vi "Temp ctrl - Read temp and stp.vi"(5 "Error In":errorcluster, 8 "Temp handle":T1={"Connected"=FALSE, "Temp ctrl"={"Gain (P)"=0.0, "Reset (I)"=0.0, "Rate (D)"=0.0, "Stabilization rate"=0.0, "Stabilization delta"=0.0, "Type"=enum."Lake Shore 325", "Custom temp ctrl"={"VISA resource name"=""}, "Lakeshore 325"={"VISA name"="", "Loop"=0, "Heater Range"=1, "Heater Resistance"=0, "Sample sensor"=0, "Fast sensor"=0, "Slow sensor"=0}, "Lakeshore 331"={"VISA name"="", "Loop"=1, "Heater Range"=0, "Sample sensor"=0, "Fast sensor"=0, "Slow sensor"=0}, "Lakeshore 332"={"VISA name"="", "Loop"=1, "Heater Range"=0, "Sample sensor"=0, "Fast sensor"=0, "Slow sensor"=0}, "Lakeshore 335"={"VISA name"="", "Loop"=1, "Sample sensor"=0, "Fast sensor"=0, "Slow sensor"=0}}} {"Temp ctrl"."Lakeshore 335"."Slow sensor" items=["A", "B"]; "Temp ctrl"."Lakeshore 335"."Fast sensor" items=["A", "B"]; "Temp ctrl"."Lakeshore 335"."Sample sensor" items=["A", "B"]; "Temp ctrl"."Lakeshore 335"."Loop" items=["Loop 1"=1, "Loop 2"=2]; "Temp ctrl"."Lakeshore 332"."Slow sensor" items=["A", "B"]; "Temp ctrl"."Lakeshore 332"."Fast sensor" items=["A", "B"]; "Temp ctrl"."Lakeshore 332"."Sample sensor" items=["A", "B"]; "Temp ctrl"."Lakeshore 332"."Heater Range" items=["Off", "Low (0.5W)", "Med (5W)", "High (50W)"]; "Temp ctrl"."Lakeshore 332"."Loop" items=["Loop 1", "Loop 2"]; "Temp ctrl"."Lakeshore 331"."Slow sensor" items=["A", "B"]; "Temp ctrl"."Lakeshore 331"."Fast sensor" items=["A", "B"]; "Temp ctrl"."Lakeshore 331"."Sample sensor" items=["A", "B"]; "Temp ctrl"."Lakeshore 331"."Heater Range" items=["Off", "Low (0.5W)", "Med (5W)", "High (50W)"]; "Temp ctrl"."Lakeshore 331"."Loop" items=["Loop 1", "Loop 2"]; "Temp ctrl"."Lakeshore 325"."Slow sensor" items=["A", "B"]; "Temp ctrl"."Lakeshore 325"."Fast sensor" items=["A", "B"]; "Temp ctrl"."Lakeshore 325"."Sample sensor" items=["A", "B"]; "Temp ctrl"."Lakeshore 325"."Heater Resistance" items=["25 Ohm"=1, "50 Ohm"=2]; "Temp ctrl"."Lakeshore 325"."Heater Range" items=["Off", "Low (loop 1) or On (loop 2)", "High (loop 1)"]; "Temp ctrl"."Lakeshore 325"."Loop" items=["Loop 1"=1, "Loop 2"=2]}) -> (0 "Error Out":errorcluster, 1 "Slow changing temp":dbl[unit], 2 "Fast changing temp":dbl[unit], 3 "Sample temperature":dbl[unit], 4 "Setpoint":dbl[unit])   [LabVIEW 2019]
doc: "Reads current temperatures and temperature setpoint from the temperature controller"
uses:
  Type defs/Temp handle Type Def.ctl
  Type defs/Temp ctrl Type Def.ctl
  Custom devices/Custom temp ctrl settings.ctl
  <instrlib>/Lake Shore 325/Public/Data/Sensor Data (Single Reading).vi
  <instrlib>/Lake Shore 335/Public/Data/Sensor Data (Single Reading).vi
  <instrlib>/Lake Shore 325/Lake Shore 325.lvlib
  <instrlib>/Lake Shore Cryotronics 331/Lake Shore Cryotronics 331.lvlib
  <instrlib>/Lake Shore Cryotronics 332/Lake Shore Cryotronics 332.lvlib
  <instrlib>/Lake Shore 335/Lake Shore 335.lvlib
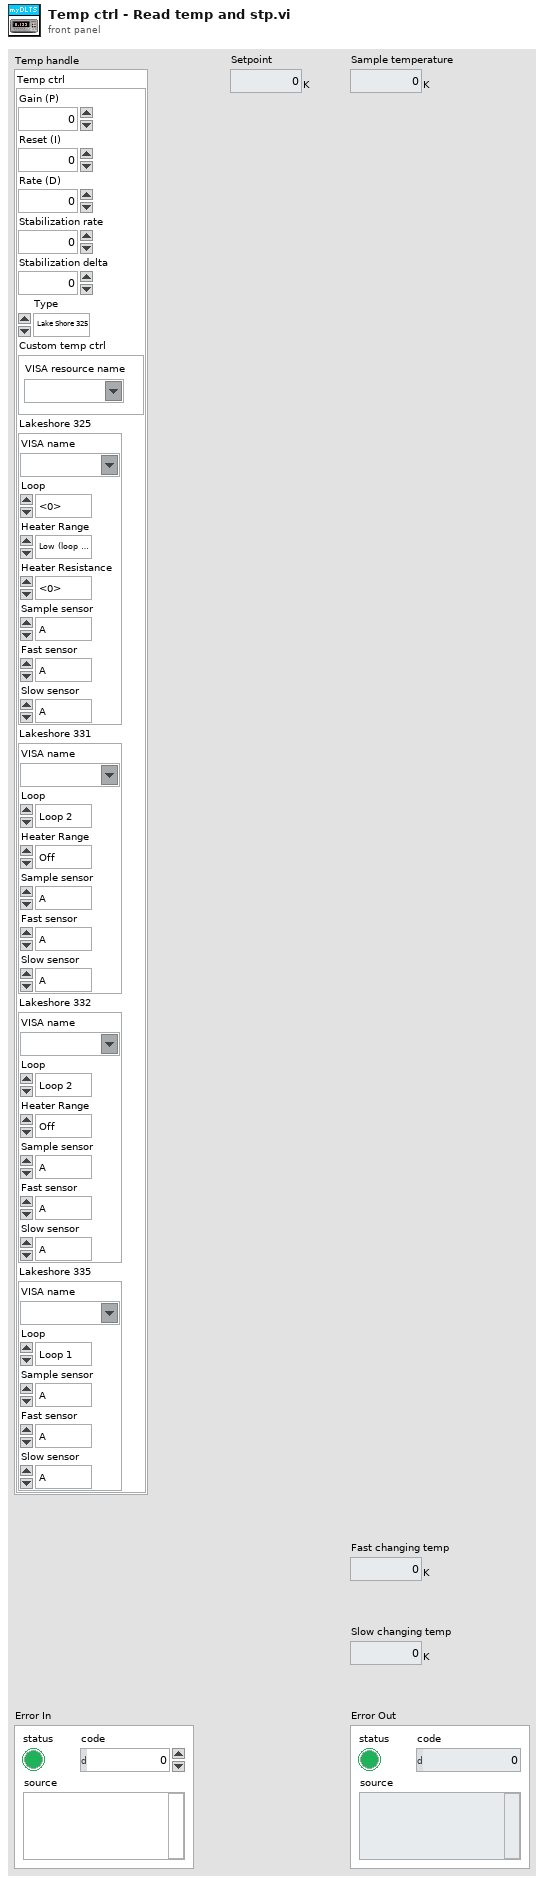
[diagram p1: front panel]
types:
  T1 = typedef "Temp handle Type Def.ctl" = cluster{"Connected":bool, "Temp ctrl":T2}
  T2 = typedef "Temp ctrl Type Def.ctl" = cluster{"Gain (P)":dbl, "Reset (I)":dbl, "Rate (D)":dbl, "Stabilization rate":dbl, "Stabilization delta":dbl, "Type":enum16{"Custom", "Lake Shore 325", "Lake Shore 331", "Lake Shore 332", "Lake Shore 335"}, "Custom temp ctrl":T3, "Lakeshore 325":cluster{"VISA name":refnum<visa-resource-name>, "Loop":u16, "Heater Range":u16, "Heater Resistance":u16, "Sample sensor":u16, "Fast sensor":u16, "Slow sensor":u16}, "Lakeshore 331":cluster{"VISA name":refnum<visa-resource-name>, "Loop":u16, "Heater Range":u16, "Sample sensor":u16, "Fast sensor":u16, "Slow sensor":u16}, "Lakeshore 332":cluster{"VISA name":refnum<visa-resource-name>, "Loop":u16, "Heater Range":u16, "Sample sensor":u16, "Fast sensor":u16, "Slow sensor":u16}, "Lakeshore 335":cluster{"VISA name":refnum<visa-resource-name>, "Loop":u16, "Sample sensor":u16, "Fast sensor":u16, "Slow sensor":u16}}
  T3 = typedef "Custom temp ctrl settings.ctl" = cluster{"VISA resource name":refnum<visa-resource-name>}
  T4 = enum16{"Custom", "Lake Shore 325", "Lake Shore 331", "Lake Shore 332", "Lake Shore 335"}
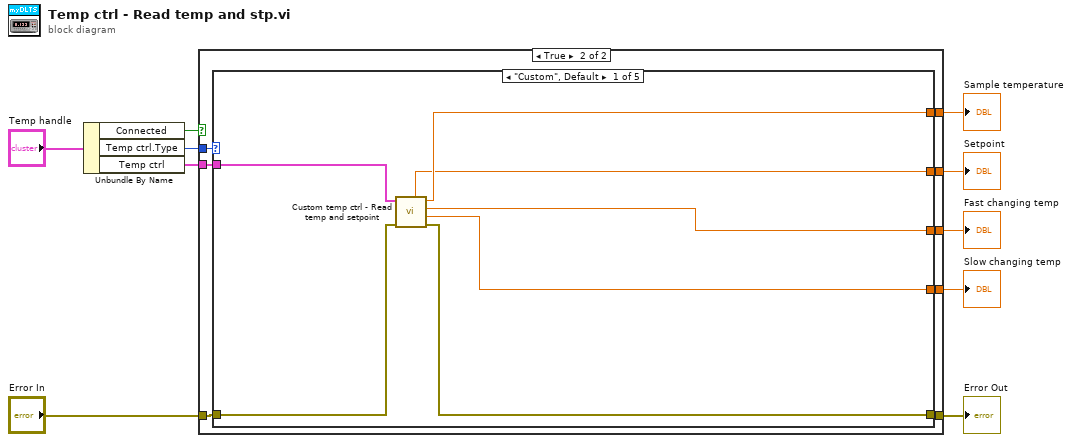
[diagram p0: block diagram]
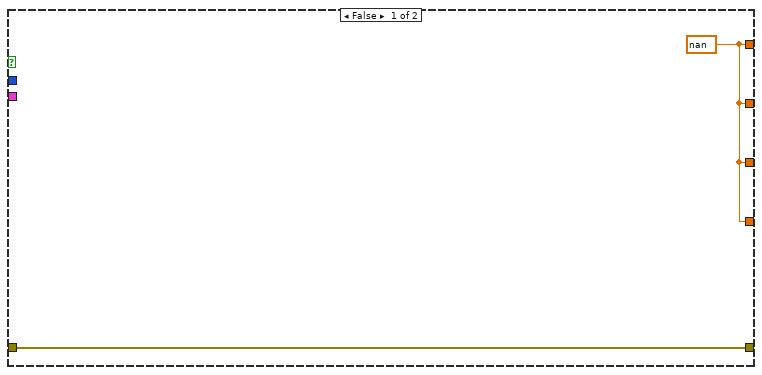
[diagram p2: hidden frame]
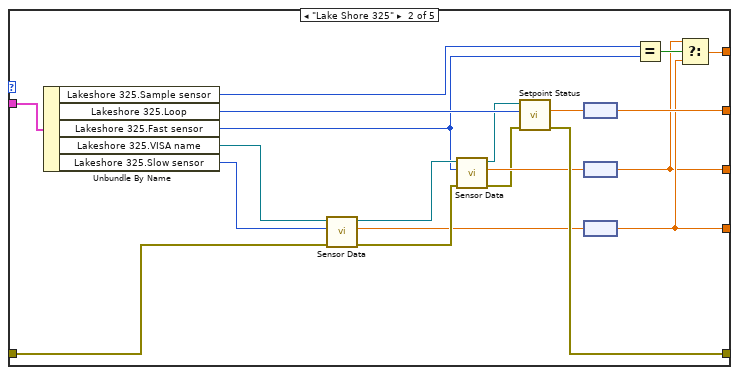
[diagram p3: hidden frame]
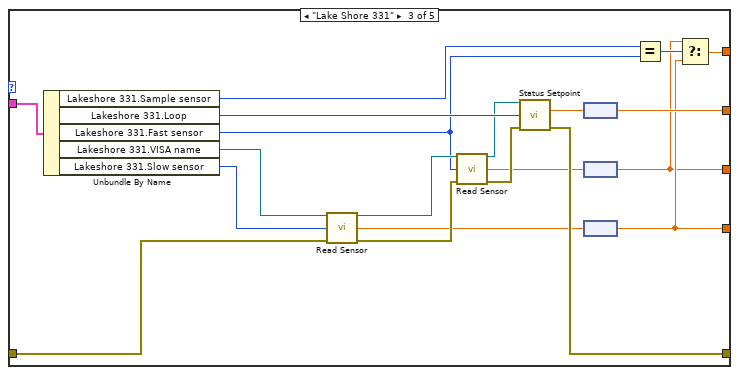
[diagram p4: hidden frame]
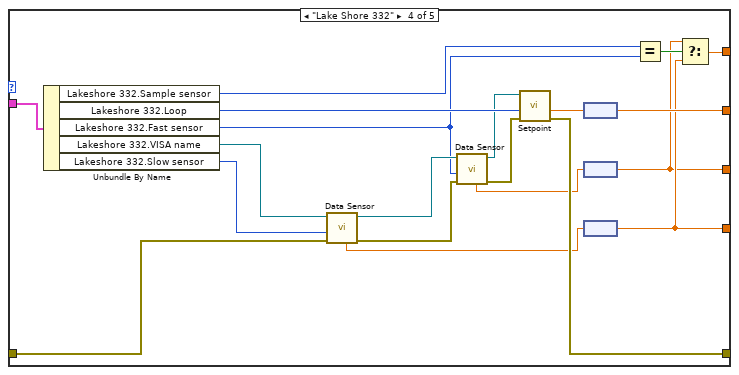
[diagram p5: hidden frame]
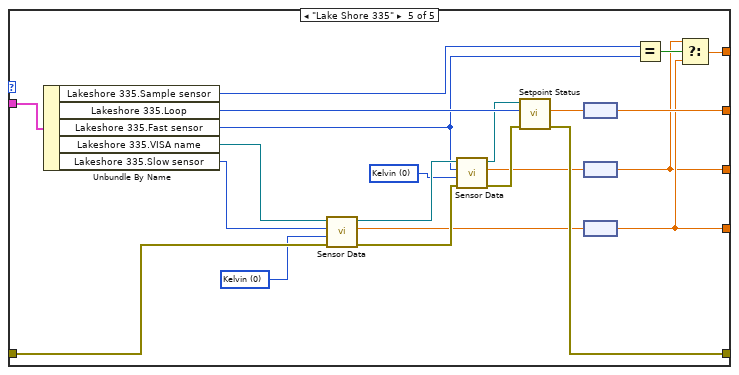
[diagram p6: hidden frame]
diagram:
  n1 = Unbundle By Name("Temp handle") -> ("Connected"=w10:bool, "Temp ctrl.Type"=w9:T4, "Temp ctrl"=w7:T2)
  n2 = case shown="True" w10 {
    tunnel: w9 -> [_ w20]
    tunnel: w7 -> [_ w19]
    tunnel: "Error In" -> [w12 w18]
    tunnel: [w12 w17] -> w5
    tunnel: [w11 w16] -> w4
    tunnel: [w11 w15] -> w3
    tunnel: [w11 w14] -> w2
    tunnel: [w11 w13] -> w1
    frame False {
      w11 = dbl[unit] nan ("Temperature")
    }
    frame True {
      n3 = case shown="\"Custom\", Default" w20 {
        tunnel: w19 -> [w26 w47 w67 w87 w109]
        tunnel: w18 -> [w27 w38 w60 w80 w102]
        tunnel: [w25 w45 w65 w85 w107] -> w17
        tunnel: [w23 w43 w63 w83 w105] -> w16
        tunnel: [w24 w32 w54 w74 w97] -> w15
        tunnel: [w22 w30 w52 w72 w95] -> w14
        tunnel: [w21 w31 w53 w73 w96] -> w13
        frame "Custom", Default {
          n4 = call "Custom temp ctrl - Read temp and setpoint.vi"("Error In"=w27, "Temp ctrl"=w26) -> ("Error Out"=w25:errorcluster, "Slow responding sensor"=w21:dbl[unit], "Fast responding sensor"=w22:dbl[unit], "Temperature"=w24:dbl[unit], "Setpoint"=w23:dbl[unit])  [unwired: 5 in]
        }
        frame "Lake Shore 325" {
          n5 = Unbundle By Name(w47) -> ("Lakeshore 325.Sample sensor"=w28:u16, "Lakeshore 325.Loop"=w46:u16, "Lakeshore 325.Fast sensor"=w29:u16, "Lakeshore 325.VISA name"=w36:refnum<visa-resource-name>, "Lakeshore 325.Slow sensor"=w37:u16)
          n6 = call-poly <instrlib>:"Sensor Data.vi"("error in (no error)"=w38, "Sensor Input (0:A)"=w37, "VISA resource name"=w36) -> ("error out"=w41:errorcluster, "Sensor Data"=w39:dbl, "VISA resource name out"=w42:refnum<visa-resource-name>)  [unwired: 6 in]
          n7 = call-poly <instrlib>:"Sensor Data.vi"("error in (no error)"=w41, "Sensor Input (0:A)"=w29, "VISA resource name"=w42) -> ("error out"=w34:errorcluster, "Sensor Data"=w40:dbl, "VISA resource name out"=w35:refnum<visa-resource-name>)  [unwired: 6 in]
          n8 = call <instrlib>:"Setpoint Status.vi"("error in (no error)"=w34, "Loop (1:Loop 1)"=w46, "VISA resource name"=w35) -> ("error out"=w45:errorcluster, "Setpoint Value"=w44:dbl)  [unwired: 6 in, 1 out]
          n9 = node(w44) -> (w43:dbl[unit])
          n10 = node(w40) -> (w30:dbl[unit])
          n11 = node(w39) -> (w31:dbl[unit])
          n12 = Equal?(x=w28, y=w29) -> (x = y?=w33:bool)
          n13 = Select(t=w30, s=w33, f=w31) -> (s? t:f=w32:dbl[unit])
        }
        frame "Lake Shore 331" {
          n14 = Unbundle By Name(w67) -> ("Lakeshore 331.Sample sensor"=w50:u16, "Lakeshore 331.Loop"=w66:u16, "Lakeshore 331.Fast sensor"=w51:u16, "Lakeshore 331.VISA name"=w58:refnum<visa-resource-name>, "Lakeshore 331.Slow sensor"=w59:u16)
          n15 = call <instrlib>:"Read Sensor.vi"("VISA resource name"=w58, "Input (0: A)"=w59, "error in (no error)"=w60) -> ("VISA resource name out"=w62:refnum<visa-resource-name>, "Kelvin Reading"=w48:dbl, "error out"=w61:errorcluster)  [unwired: 8 in, 2 out]
          n16 = call <instrlib>:"Read Sensor.vi"("VISA resource name"=w62, "Input (0: A)"=w51, "error in (no error)"=w61) -> ("VISA resource name out"=w57:refnum<visa-resource-name>, "Kelvin Reading"=w49:dbl, "error out"=w56:errorcluster)  [unwired: 8 in, 2 out]
          n17 = call <instrlib>:"Status Setpoint.vi"("VISA resource name"=w57, "Loop (0: 1)"=w66, "error in (no error)"=w56) -> ("Setpoint"=w64:dbl, "error out"=w65:errorcluster)  [unwired: 10 in, 1 out]
          n18 = node(w64) -> (w63:dbl[unit])
          n19 = node(w49) -> (w52:dbl[unit])
          n20 = node(w48) -> (w53:dbl[unit])
          n21 = Equal?(x=w50, y=w51) -> (x = y?=w55:bool)
          n22 = Select(t=w52, s=w55, f=w53) -> (s? t:f=w54:dbl[unit])
        }
        frame "Lake Shore 332" {
          n23 = Unbundle By Name(w87) -> ("Lakeshore 332.Sample sensor"=w70:u16, "Lakeshore 332.Loop"=w86:u16, "Lakeshore 332.Fast sensor"=w71:u16, "Lakeshore 332.VISA name"=w78:refnum<visa-resource-name>, "Lakeshore 332.Slow sensor"=w79:u16)
          n24 = call <instrlib>:"Data Sensor.vi"("error in (no error)"=w80, "Input (0: A)"=w79, "VISA resource name"=w78) -> ("error out"=w81:errorcluster, "VISA resource name out"=w82:refnum<visa-resource-name>, "Kelvin Reading"=w69:dbl)  [unwired: 4 in, 2 out]
          n25 = call <instrlib>:"Data Sensor.vi"("error in (no error)"=w81, "Input (0: A)"=w71, "VISA resource name"=w82) -> ("error out"=w76:errorcluster, "VISA resource name out"=w77:refnum<visa-resource-name>, "Kelvin Reading"=w68:dbl)  [unwired: 4 in, 2 out]
          n26 = call <instrlib>:"Setpoint.vi"("error in (no error)"=w76, "Loop (0: 1)"=w86, "VISA resource name"=w77) -> ("error out"=w85:errorcluster, "Setpoint"=w84:dbl)  [unwired: 6 in, 1 out]
          n27 = node(w84) -> (w83:dbl[unit])
          n28 = node(w68) -> (w72:dbl[unit])
          n29 = node(w69) -> (w73:dbl[unit])
          n30 = Equal?(x=w70, y=w71) -> (x = y?=w75:bool)
          n31 = Select(t=w72, s=w75, f=w73) -> (s? t:f=w74:dbl[unit])
        }
        frame "Lake Shore 335" {
          w88 = u16 0 items=["Kelvin", "Celsius", "Sensor Units"] ("Data Source (0:Kelvin)")
          w90 = u16 0 items=["Kelvin", "Celsius", "Sensor Units"] ("Data Source (0:Kelvin)")
          n32 = Unbundle By Name(w109) -> ("Lakeshore 335.Sample sensor"=w94:u16, "Lakeshore 335.Loop"=w108:u16, "Lakeshore 335.Fast sensor"=w91:u16, "Lakeshore 335.VISA name"=w101:refnum<visa-resource-name>, "Lakeshore 335.Slow sensor"=w89:u16)
          n33 = call-poly <instrlib>:"Sensor Data.vi"("error in (no error)"=w102, "Data Source (0:Kelvin)"=w88, "Input (0:A)"=w89, "VISA resource name"=w101) -> ("error out"=w103:errorcluster, "Sensor Data"=w93:dbl, "VISA resource name out"=w104:refnum<visa-resource-name>)  [unwired: 5 in]
          n34 = call-poly <instrlib>:"Sensor Data.vi"("error in (no error)"=w103, "Data Source (0:Kelvin)"=w90, "Input (0:A)"=w91, "VISA resource name"=w104) -> ("error out"=w99:errorcluster, "Sensor Data"=w92:dbl, "VISA resource name out"=w100:refnum<visa-resource-name>)  [unwired: 5 in]
          n35 = call <instrlib>:"Setpoint Status.vi"("error in (no error)"=w99, "Output (1:1)"=w108, "VISA resource name"=w100) -> ("error out"=w107:errorcluster, "Setpoint"=w106:dbl)  [unwired: 6 in, 1 out]
          n36 = node(w106) -> (w105:dbl[unit])
          n37 = node(w92) -> (w95:dbl[unit])
          n38 = node(w93) -> (w96:dbl[unit])
          n39 = Equal?(x=w94, y=w91) -> (x = y?=w98:bool)
          n40 = Select(t=w95, s=w98, f=w96) -> (s? t:f=w97:dbl[unit])
        }
      }
    }
  }
  "Error Out" <- w5
  "Setpoint" <- w4
  "Sample temperature" <- w3
  "Slow changing temp" <- w1
  "Fast changing temp" <- w2
